vi "Disconnect.vi"(8 "Error In":errorcluster, 10 "Resource Name":refnum<k15>, 11 "object in":refnum<class "Connected.lvclass">) -> (0 "Error Out":errorcluster, 3 "object out":refnum<class "IStates.lvclass">)   [LabVIEW 2023, in "PXI-5441.lvlib" / "Connected.lvclass"]
uses:
  Connected.lvclass
  IScope_interface/IStates_interface/IStates.lvclass
  Disconnected_class/Disconnected.lvclass
  Connected.lvclass/Connected.ctl
  D:/git/HAL/PXI-5441_class/states/Disconnected_class/Disconnected.lvclass
  D:/git/HAL/IScope_interface/IStates_interface/IStates.lvclass
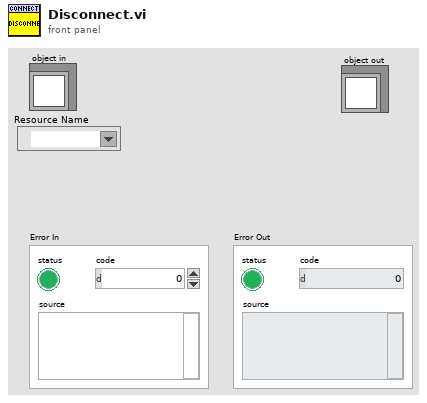
[diagram p1: front panel]
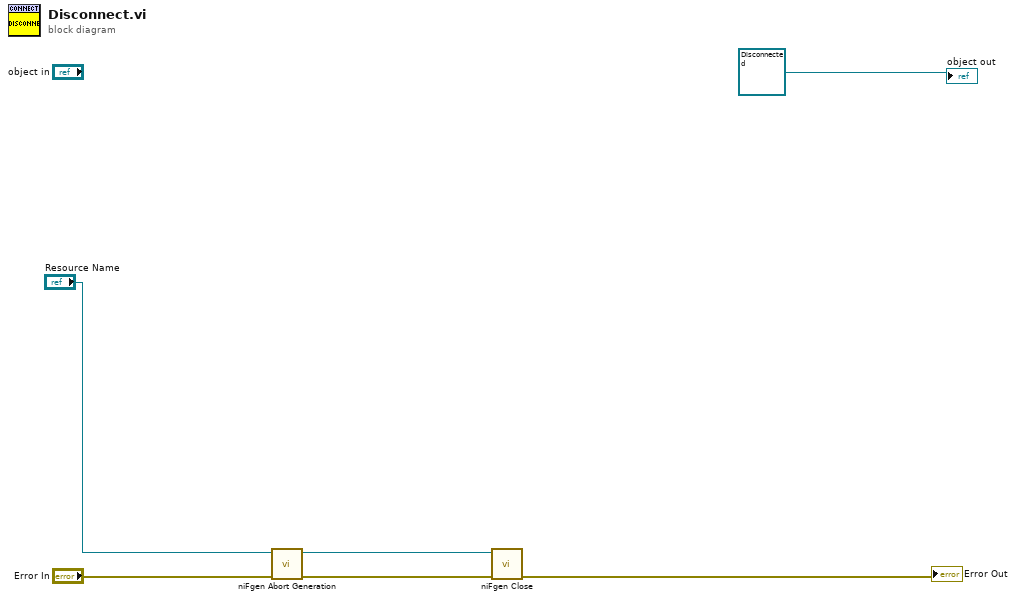
[diagram p0: block diagram]
diagram:
  n1 = call <instrlib>:"niFgen Abort Generation.vi"("error in (no error)"="Error In", "Instrument Handle"="Resource Name") -> ("error out"=w4:errorcluster, "Instrument Handle Out"=w2:refnum<k15>)  [unwired: 8 in]
  n2 = call <instrlib>:"niFgen Close.vi"("error in (no error)"=w4, "Instrument Handle"=w2) -> ("error out"=→"Error Out":errorcluster)  [unwired: 9 in]
  "object out" <- refnum<class "Disconnected.lvclass"> refnum ("PXI-5441.lvlib:Disconnected")
